vi "Constrain Log Size.vi"(11 "Debug Log in":refnum<class "Debug Log.lvclass">) -> (3 "Debug Log out":refnum<class "Debug Log.lvclass">)   [LabVIEW 2020, in "Debug Log.lvclass"]
uses:
  Debug Log.lvclass
  Debug Log.lvclass/Debug Log.ctl
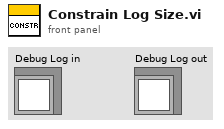
[diagram p1: front panel]
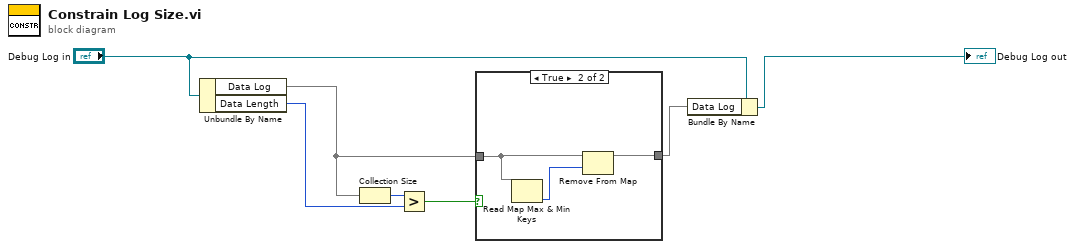
[diagram p0: block diagram]
diagram:
  n1 = Unbundle By Name("Debug Log in") -> ("Data Log"=w4:map{u32, refnum<class "Debug Data.lvclass">}, "Data Length"=w2:i32)
  n2 = Collection Size(1:w4) -> (0:w1:i32)
  n3 = Greater?(x=w1, y=w2) -> (0:w3:bool)
  n4 = case shown="True" w3 {
    tunnel: w4 -> [w8 w11]
    tunnel: [w8 w9] -> w6
    frame False {
    }
    frame True {
      n5 = Read Map Max & Min Keys(11:w11) -> (1:w10:u32)  [unwired: 1 out]
      n6 = Remove From Map(10:w10, 11:w11) -> (3:w9:map{u32, refnum<class "Debug Data.lvclass">})  [unwired: 2 out]
    }
  }
  n7 = Bundle By Name(cluster="Debug Log in", "Data Log"=w6) -> (→"Debug Log out":refnum<class "Debug Log.lvclass">)
